vi "Dashboard Main.vi"() -> ()   [LabVIEW 2012]
uses:
  <vilib>/Utility/miscctls.llb/LVRectTypeDef.ctl
  <vilib>/event_ctls.llb/eventvkey.ctl
  <vilib>/Utility/config.llb/Read Key (String).vi
  <vilib>/Utility/config.llb/Read Key (I32).vi
  <vilib>/Utility/config.llb/Write Key (String).vi
  <vilib>/Utility/config.llb/Write Key (I32).vi
  <vilib>/Rock Robotics/Network Tables/SD Write Number.vi
  <vilib>/Rock Robotics/Network Tables/SD Read Number.vi
  <vilib>/Rock Robotics/Network Tables/SD Read Boolean.vi
  <vilib>/Utility/config.llb/NI_LVConfig.lvlib
panel:
  out "Predicted Y Coordionates":sgl
  in  "Camera Settings":T1={"Frate Rate"=10, "Compression"=39, "Size"=1} {"Frate Rate" scale=1.0..30.0; "Size" items=["640x480", "320x240", "160x120"]}
  out "Mode":T2(ring)=enum.""
  out "Camera IP":string="0.0.0.11"
  in  "Dashboard Tab":T3(tab)=enum."Normal Operation"
  out "High Y":dbl
  in  "Red or Hue":cluster{"Lower value":i32, "Upper value":i32}={"Lower value"=52, "Upper value"=255}
  in  "Green or Sat":cluster{"Lower value":i32, "Upper value":i32}={"Lower value"=80, "Upper value"=255}
  in  "Blue or Luma or Val or Inten":cluster{"Lower value":i32, "Upper value":i32}={"Lower value"=80, "Upper value"=255}
  in  "Turn On Vision":bool=TRUE
  out "Vision Working?":bool=TRUE
  out "High Y String":string
  out "Predicted X":sgl
  in  "Crosshair":bool=TRUE
  out "Camera Image 2":T4(plugin-control)
  out "Lines (Shape Detection 1)":T5(array[cluster]) {"End Point"."Y" format="%.2f"; "End Point"."X" format="%.2f"; "Start Point"."Y" format="%.2f"; "Start Point"."X" format="%.2f"}
  in  "Assisted Vision":bool=TRUE
  in  "Blackout":bool=TRUE
  in  "Slider":dbl(slide) scale=0.0..100.0 scale format="%#_3g"
  in  "On/Off":bool caption="Solenoid"
  in  "Test Name":u16(ring) items=["Select the test to run...", "Example Test", "-------------------------------", "List of tests is built in robot code.", "Replace with your own automated tests."]
  in  "Test Tree":string(tree)
  in  "Motor":cluster{"Value":dbl, "Enable":bool} {"Value" scale=-1.0..1.0 scale format="%#_3g"}
  out "Progress":T6 {"Test Progress" scale=0.0..100.0}
  in  "Rev/Fwd":cluster{"Forward":bool, "Reverse":bool}
  in  "Ring":u16(ring) items=["Auto", "Fixed indoor", "Fixed outdoor 1", "Fixed outdoor 2", "Fixed fluorescent 1", "Fixed fluorescent 2", "Hold current"]
  in  "Listbox":i32(listbox)
  out "MotorSlide4":dbl(slide) scale=-1.0..1.0 scale format="%#_2e"
  out "MotorSlide3":dbl(slide) scale=-1.0..1.0 scale format="%#_2e"
  out "MotorSlide2":dbl(slide) scale=-1.0..1.0 scale format="%#_2e"
  in  "MotorName3":string="Front Left"
  in  "MotorName4":string="Front Right"
  in  "MotorName1":string="Rear Left"
  in  "MotorName2":string="Rear Right"
  out "MotorChart4":dbl(graph)
  out "MotorChart3":dbl(graph)
  out "MotorChart2":dbl(graph)
  out "MotorSlide1":dbl(slide) scale=-1.0..1.0 scale format="%#_2e"
  out "MotorChart1":dbl(graph)
  out "JS1 Z":dbl(slide) scale=-1.0..1.0 scale format="%#_2e"
  out "JS2 Z":dbl(slide) scale=-1.0..1.0 scale format="%#_2e"
  out "Joystick 1":cluster{"X":dbl, "Y":dbl}[](graph)
  out "Joystick 2":cluster{"X":dbl, "Y":dbl}[](graph)
  out "JS Buttons 1":T7
  out "JS Buttons 2":T7
  out "Robot IP":string="0.0.0.0"
  out "Battery Value":dbl(slide) scale=0.0..14.0 scale format="%#_2e"
  out "Battery":sgl(graph)
  out "Vision Locked On":bool
  out "Upper LED":bool
  out "Lower LED":bool
  out "Shooter RPM":dbl(slide) scale=0.0..12000.0
  out "Shooter Rotation Angle":dbl(knob) scale=0.0..90.0
  out "Up to Speed?":bool
  out "SHOOT!":bool
  out "Angle":dbl
  in  "Viewer":T8(tab)
  out "Mbps":dbl format="%#.1g"
  in  "Enable":bool=TRUE
  in  "DB Camera Config":bool
  out "Mbps":bool
  out "fps":dbl format="%#.1g"
  out "Image Error Message":string="Timeout in Camera Communications"
  out "Camera Image":T4(plugin-control)
  out "Camera Image 3":T4(plugin-control)
  out "Buttons 1":cluster{"1":bool, "2":bool, "3":bool}
  out "Kinect 1":cluster{"X":dbl, "Y":dbl, "Z":dbl} {"X" scale=1.0..-1.0; "Y" scale=1.0..-1.0; "Z" scale=1.0..-1.0}
  out "Buttons 2":cluster{"1":bool, "2":bool, "3":bool}
  out "Kinect 2":cluster{"X":dbl, "Y":dbl, "Z":dbl} {"X" scale=1.0..-1.0; "Y" scale=1.0..-1.0; "Z" scale=1.0..-1.0}
  out "Version":string
  out "Skeleton Picture":picture
  out "Players":i8
  out "Tree":string(tree)
  # "http://team223.com/Images/TopPane/spinning-gear.gif"
  # "Drive & Motors"
  # "Robot IP:"
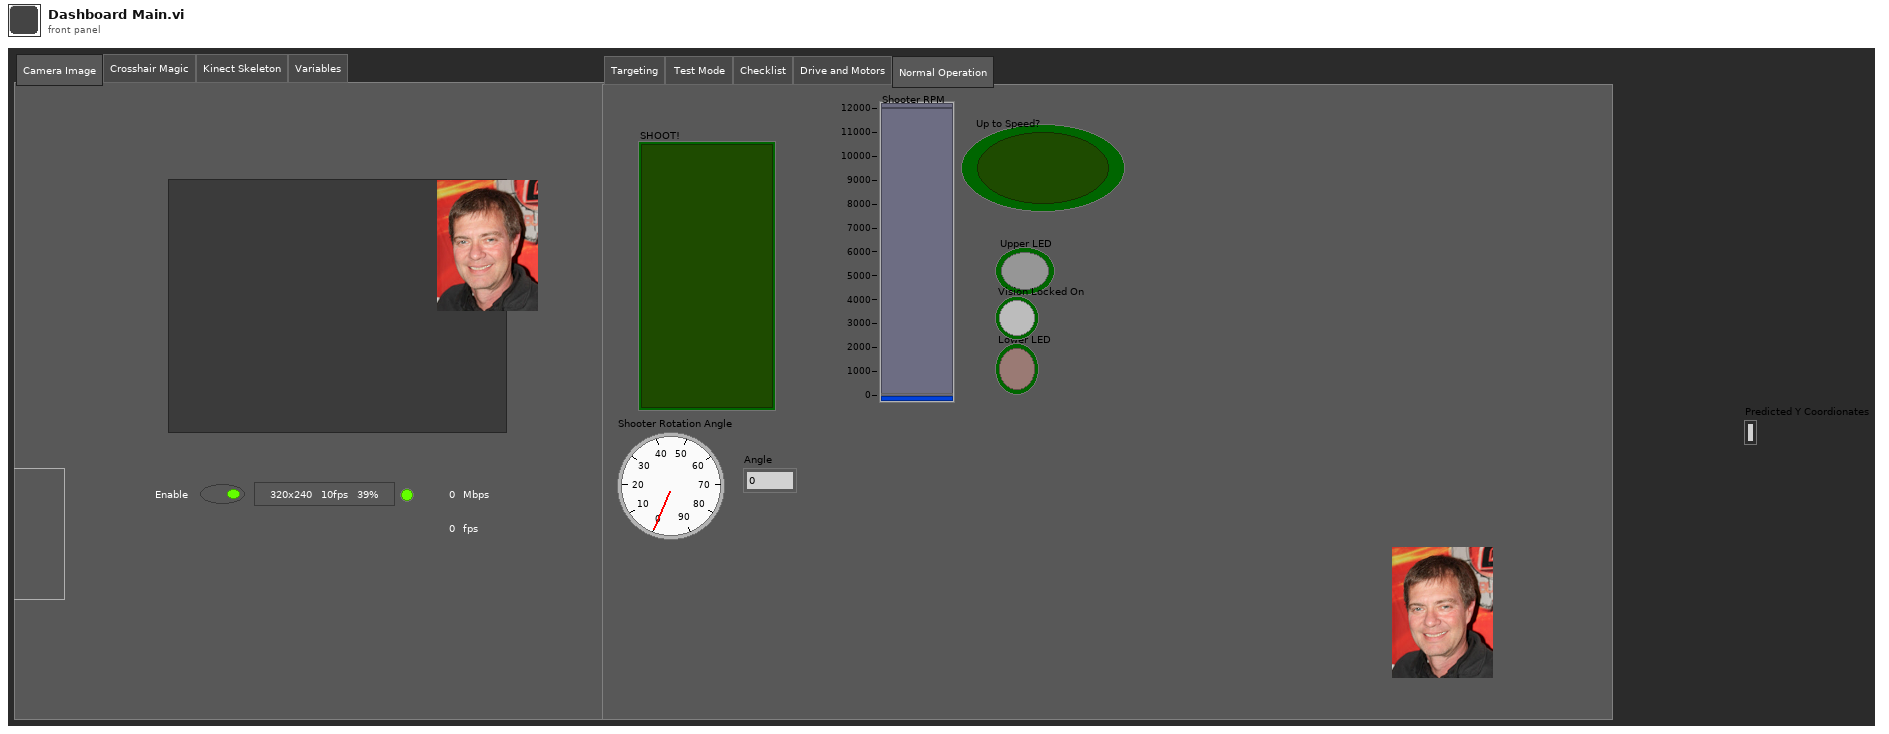
[diagram p1: front panel]
types:
  T1 = cluster{"Frate Rate":i32, "Compression":i32, "Size":u16}
  T2 = enum8{"Tele-Op Disabled", "Tele-Op Enabled", "Auto Disabled", "Auto Enabled", "Test Disabled", "Test Enabled", ""}
  T3 = enum32{"Targeting", "Test Mode ", "Checklist", "Drive and Motors", "Normal Operation"}
  T4 = typedef "IMAQ Image.ctl" = refnum<image>
  T5 = cluster{"Start Point":cluster{"X":sgl, "Y":sgl}, "End Point":cluster{"X":sgl, "Y":sgl}, "Length":dbl, "Orientation":dbl, "Score":dbl}[]
  T6 = cluster{"Test Progress":u8, "Test Progress Text":string}
  T7 = cluster{bool, bool, bool, bool, bool, bool, bool, bool, bool, bool, bool, bool}
  T8 = enum32{"Camera Image", "Crosshair Magic", "Kinect Skeleton", "Variables"}
  T9 = typedef "Image Type" = u32
  T10 = typedef "LVBoundsTypeDef.ctl" = cluster{"Width":u32, "Height":u32}
  T11 = typedef "SkeletonTrackState.ctl" = enum32{"NotTracked", "PositionOnly", "Tracked"}
  T12 = cluster{"TrackingState":u8[], "Position":cluster{"x":sgl, "y":sgl, "z":sgl}, cluster{"x":sgl, "y":sgl, "z":sgl, sgl}[], "TrackState":T11}
  T13 = cluster{cluster{"ScaledToPercentRange":dbl, "ScaledToPercentRange":dbl, "ScaledToPercentRange":dbl}, cluster{bool, bool, bool}}[]
  T14 = cluster{cluster{"ScaledToPercentRange":dbl, "ScaledToPercentRange":dbl, "ScaledToPercentRange":dbl}, cluster{bool, bool, bool}}
  T15 = cluster{"ScaledToPercentRange":dbl, "ScaledToPercentRange":dbl, "ScaledToPercentRange":dbl}
  T16 = typedef "LVRectTypeDef.ctl" = cluster{"Left":i16, "Top":i16, "Right":i16, "Bottom":i16}
  T17 = cluster{"Left":i32, "Top":i32, "Right":i32, "Bottom":i32}
  T18 = cluster{"Competition mode":bool, "Robot Link":bool, "Autonomous":bool, "Enabled":bool, "E-Stop":bool, "Simulated":bool, "TestMode":bool, "Docked Window":bool}
  T19 = cluster{"Boolean Array[0]":bool, "Boolean Array[1]":bool, "Boolean Array[2]":bool, "Boolean Array[3]":bool, "Boolean Array[4]":bool, "Boolean Array[5]":bool, "Boolean Array[6]":bool, "Boolean Array[7]":bool, "Boolean Array[8]":bool, "Boolean Array[9]":bool, "Boolean Array[10]":bool, "Boolean Array[11]":bool}
  T20 = typedef "NI_LVConfig.lvlib/Config Data RefNum.ctl" = refnum<k1>
  T21 = cluster{"Boolean array[0]":bool, "Boolean array[1]":bool, "Boolean array[2]":bool, "Boolean array[3]":bool, "Boolean array[4]":bool, "Boolean array[5]":bool, "Boolean array[6]":bool, "Boolean array[7]":bool, "Boolean array[8]":bool}
  T22 = typedef "eventvkey.ctl" = enum16{"ASCII", "Enter", "Return", "Shift", "Ctrl", "Alt", "Cmd", "Opt", "Caps", "NumLock", "Clear", "Break", "Up", "Down", "Left", "Right", "Insert", "Delete", "Home", "End", "PageUp", "PageDown", "Escape", "Help", "Pause", "ScrollLock", "F1", "F2", "F3", "F4", "F5", "F6", "F7", "F8", "F9", "F10", "F11", "F12", "F13", "F14", "F15", "F16", "F17", "F18", "F19", "F20", "F21", "F22", "F23", "F24", "Play", "VolumeUp", "VolumeDown", "Mute", "Two Byte Char"}
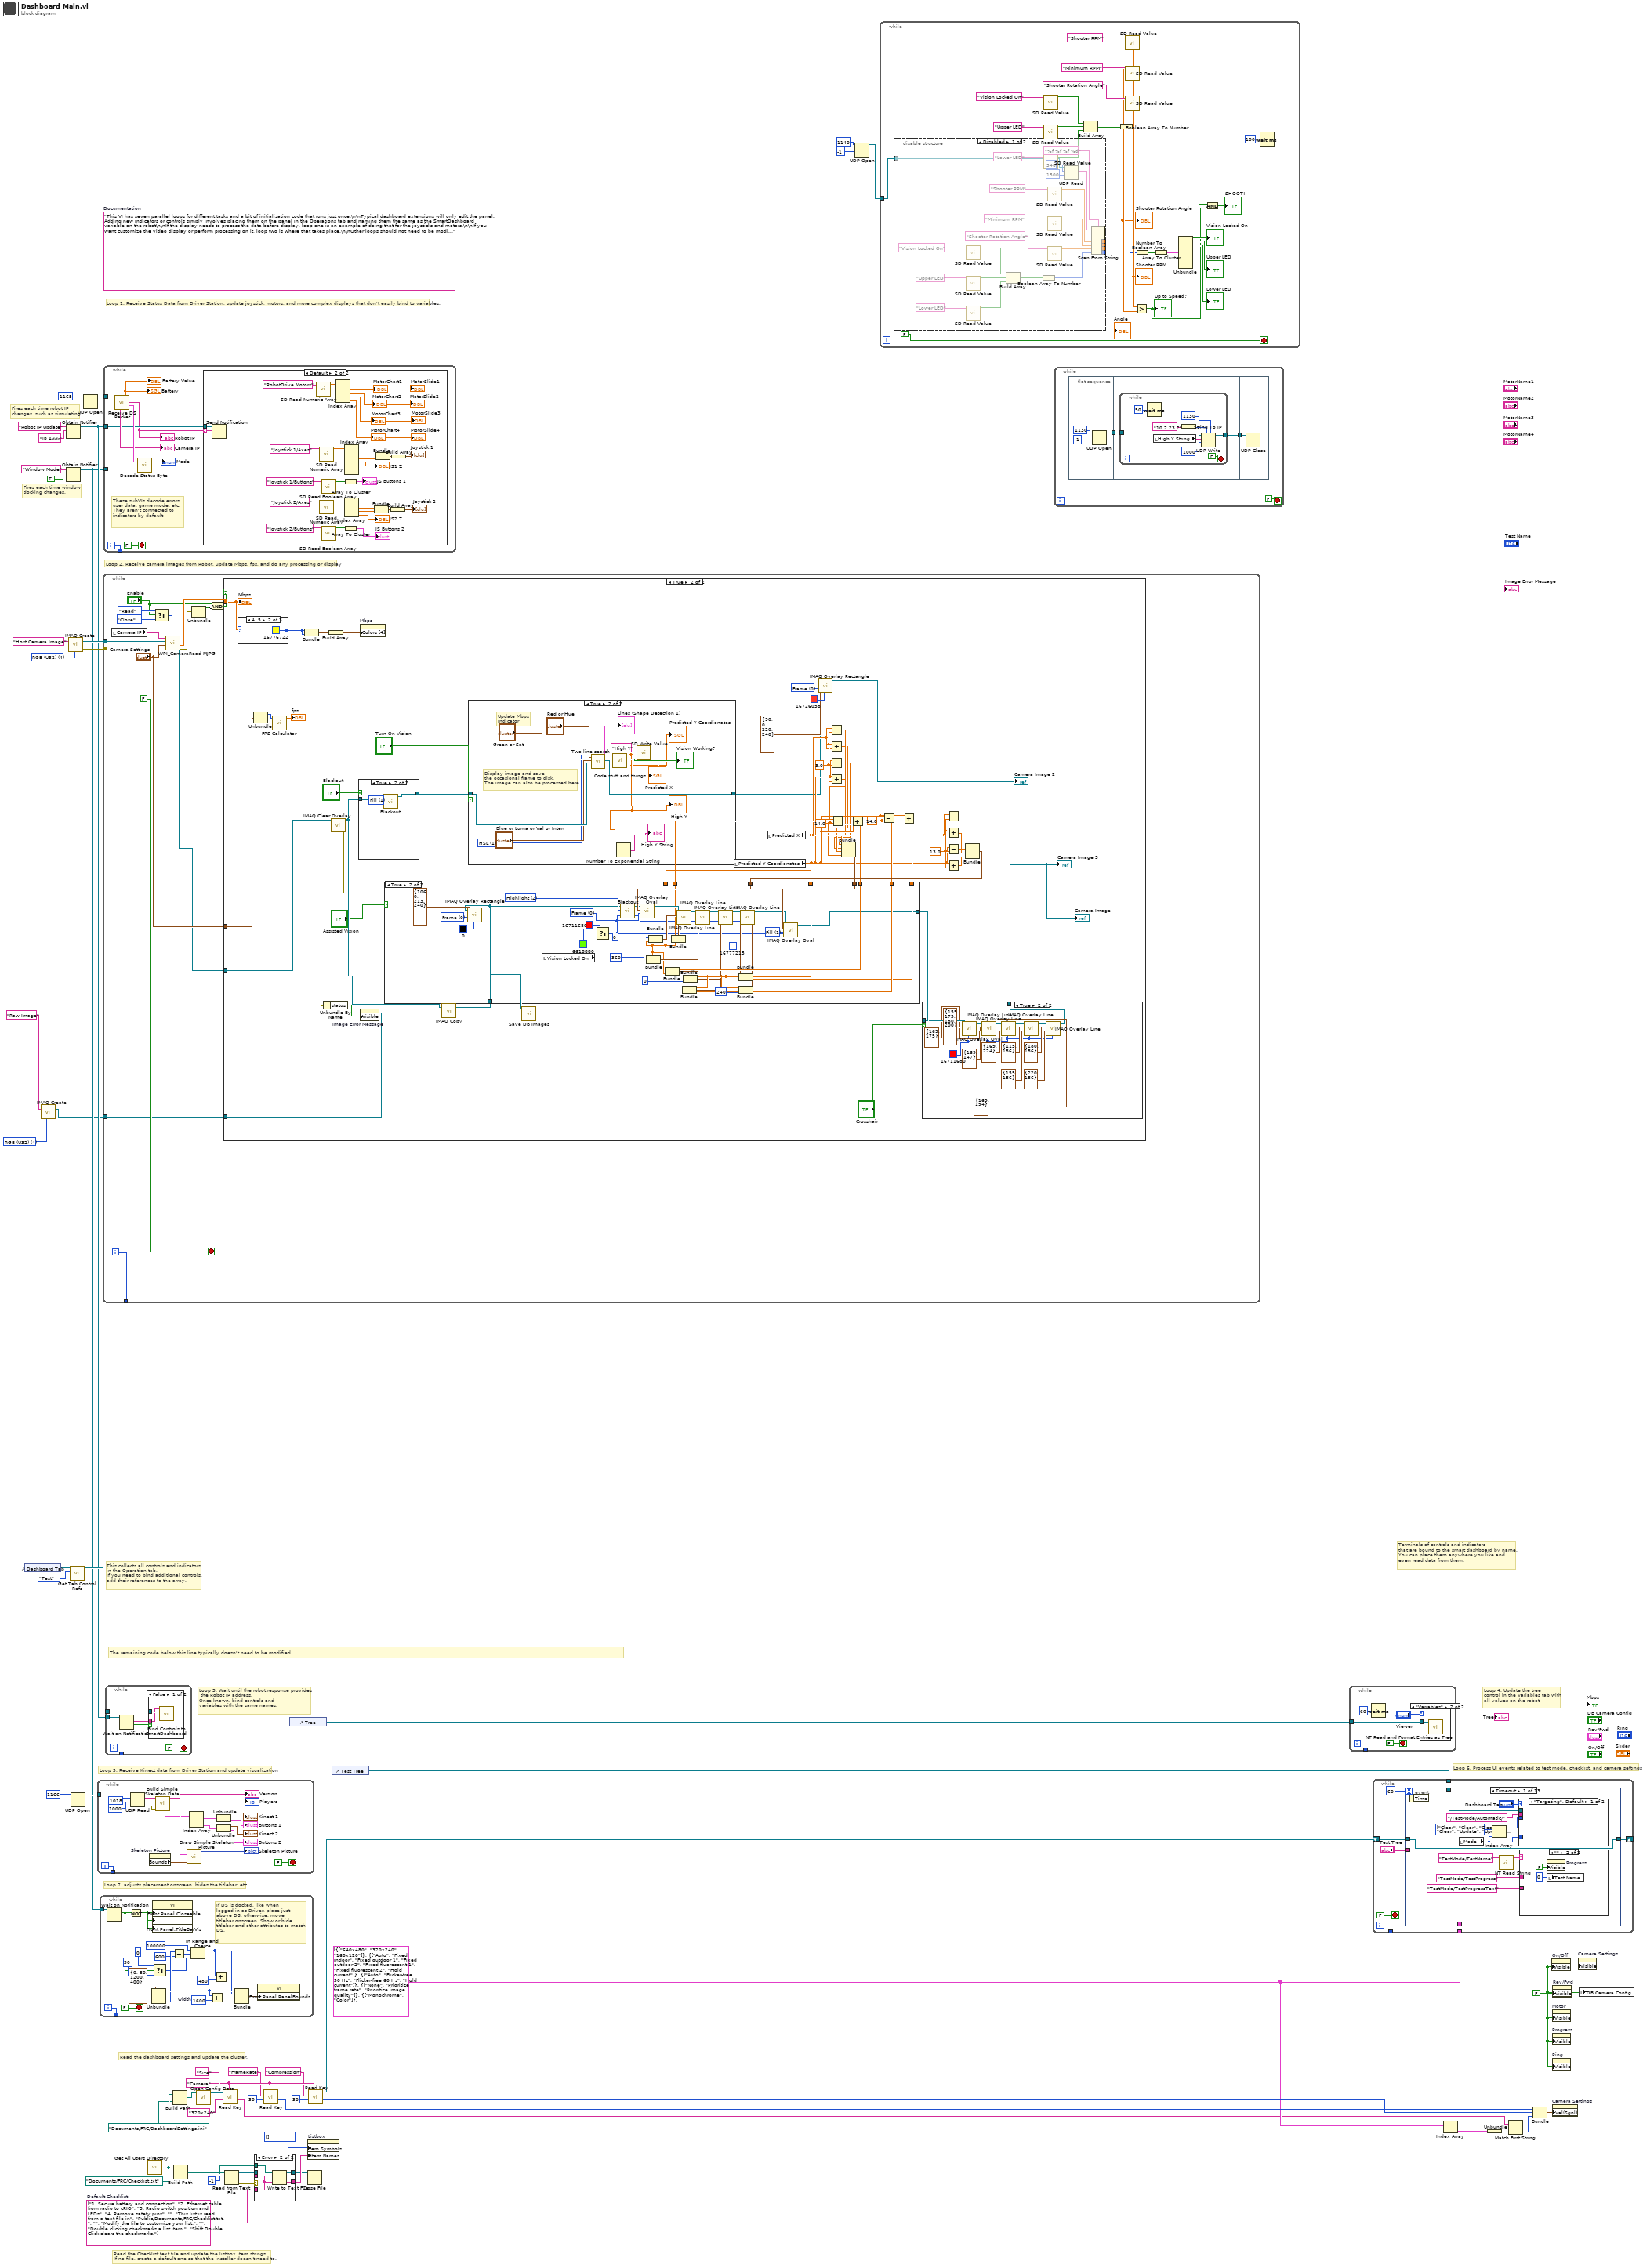
[diagram p0: block diagram]
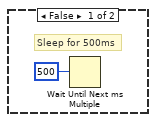
[diagram p4: hidden frame]
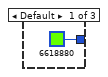
[diagram p9: hidden frame]
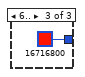
[diagram p10: hidden frame]
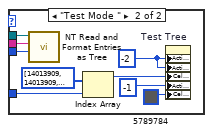
[diagram p12: hidden frame]
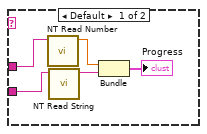
[diagram p13: hidden frame]
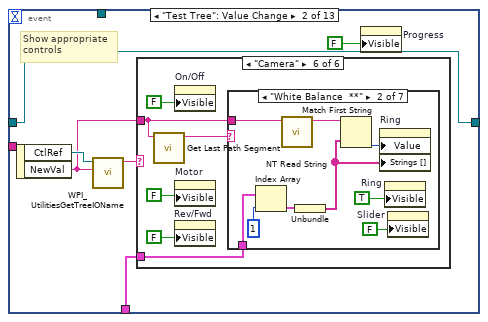
[diagram p14: hidden frame]
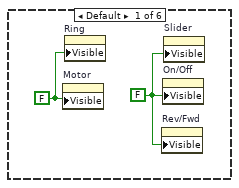
[diagram p15: hidden frame]
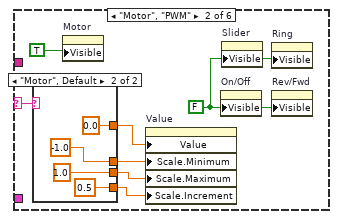
[diagram p16: hidden frame]
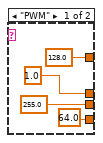
[diagram p17: hidden frame]
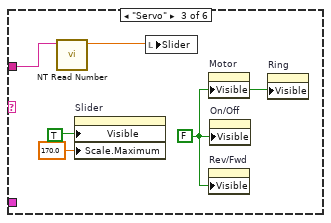
[diagram p18: hidden frame]
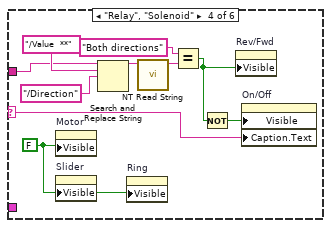
[diagram p19: hidden frame]
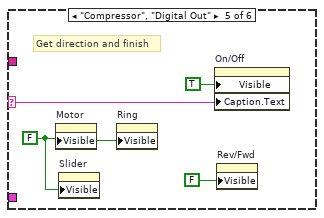
[diagram p20: hidden frame]
diagram:
  w6 = T9 4 items=["Grayscale (U8)", "Grayscale (I16)", "Grayscale (SGL)", "Complex (CSG)", "RGB (U32)", "HSL (U32)", "RGB (U64)"] ("Image Type")
  w27 = "Camera"
  w19 = cluster{string[]}[] [{["640x480", "320x240", "160x120"]}, {["Auto", "Fixed indoor", "Fixed outdoor 1", "Fixed outdoor 2", "Fixed fluorescent 1", "Fixed fluorescent 2", "Hold current"]}, {["Auto", "Flicker-free 50 Hz", "Flicker-free 60 Hz", "Hold current"]}, {["None", "Prioritize frame rate", "Prioritize image quality"]}, {["Monochrome", "Color"]}]
  w35 = string[] ["1. Secure battery and connection", "2. Ethernet cable from radio to cRIO", "3. Radio switch position and LEDs", "4. Remove safety pins", "", "This list is read from a text file in", "Public/Documents/FRC/Checklist.txt.", "", "Modify the file to customize your list.", "", "Double clicking checkmarks a list item.", "Shift Double Click clears the checkmarks."]  # Default Checklist
  w33 = FALSE ("Visible")
  (unwired) "This VI has seven parallel loops for different tasks and a bit of initialization code that runs just once.\n\nTypical dashboard extensions will only edit the panel. Adding new indicators or controls simply involves placing them on the panel in the Operations tab and naming them the same as the SmartDashboard variable on the robot\n\nIf the display needs to process the data before display, loop one is an example of doing that for the joysticks and motors.\n\nIf you want customize the video display or perform processing on it, loop two is where that takes place.\n\nOther loops should not need to be modified. They are pretty standard, and document the task they perform."  # Documentation
  w56 = T9 4 items=["Grayscale (U8)", "Grayscale (I16)", "Grayscale (SGL)", "Complex (CSG)", "RGB (U32)", "HSL (U32)", "RGB (U64)"] ("Image Type")
  # "Fires each time robot IP\nchanges, such as simulating"
  # "Fires each time window\ndocking changes."
  # "Read the Checklist text file and update the listbox item strings.\nIf no file, create a default one so that the installer doesn't need to."
  # "This collects all controls and indicators\nin the Operation tab.\nIf you need to bind additional controls,\nadd their references to the array."
  # "The remaining code below this line typically doesn't need to be modified."
  # "Loop 6. Process UI events related to test mode, checklist, and camera settings"
  # "Read the dashboard settings and update the cluster."
  # "Terminals of controls and indicators\nthat are bound to the smart dashboard by name.\nYou can place them anywhere you like and\neven read data from them."
  # "Loop 4. Update the tree\ncontrol in the Variables tab with\nall values on the robot"
  # "Loop 3. Wait until the robot response provides\n the Robot IP address.\nOnce known, bind controls and\nvariables with the same names."
  # "Loop 5. Receive Kinect data from Driver Station and update visualization"
  # "Loop 7. adjusts placement onscreen, hides the titlebar, etc."
  # "Loop 1. Receive Status Data from Driver Station, update joystick, motors, and more complex displays that don't easily bind to variables."
  # "Loop 2. Receive camera images from Robot, update Mbps, fps, and do any processing or display"
  n1 = control-ref of="Dashboard Tab"() -> (w49:refnum<vi>)
  n2 = call "IMAQ Create"("Image Name"="Raw Image", "Image Type"=w6) -> ("New Image"=w4:T4)  [unwired: 2 in, 2 out]
  n3 = Obtain Notifier(name (unnamed)="Robot IP Update", notification data type="IP Addr" ("name (unnamed)")) -> (notifier out=w46:refnum<notifier>)  [unwired: 2 in, 2 out]
  n4 = Obtain Notifier(name (unnamed)="Window Mode", notification data type=TRUE) -> (notifier out=w39:refnum<notifier>)  [unwired: 2 in, 2 out]
  n5 = call "IMAQ Create"("Image Name"="Host Camera Image", "Image Type"=w56) -> ("New Image"=w54:T4, "error out"=w53:errorcluster)  [unwired: 2 in, 1 out]
  n6 = call <vilib>:"Get Tab Control Refs.vi"("Page Index"=enum32{"Operation", "Test"}."Test" ("Dashboard Tab"), "TabControl in"=w49) -> ("ControlsOnPage"=w50:refnum<vi>[])  [unwired: 9 in]
  n7 = UDP Open(11:u16 1166 ("port")) -> (port=w51:refnum<k16>)  [unwired: 2 in, 4 out]
  n8 = UDP Open(11:u16 1165 ("port")) -> (port=w57:refnum<k16>)  [unwired: 2 in, 4 out]
  n9 = while {
    tunnel: w51 -> [w75]
    tunnel: [w60] -> _
    i -> [w60]
    stop <- FALSE stop-if-true
    n10 = UDP Read(connection ID=w75, max size (548)=1018 ("bytes to read"), timeout ms (25000)=1000) -> (data out=w69:string, error out=w59:errorcluster)  [unwired: 1 in, 3 out]
    n11 = property on="Skeleton Picture" class="Pict"() -> ("Bounds"=w71:T10)  [unwired: 2 in, 2 out]
    n12 = call "Build Simple Skeleton Data.vi"("error in (no error)"=w59, "data in"=w69) -> ("Skeleton Data"=w70:T12, "NumPlayers"=→"Players":i8, "Version String"=→"Version":string, "Simple Joystick Info"=w67:T13)  [unwired: 5 in, 1 out]
    n13 = call "Draw Simple Skeleton Picture.vi"("Bounds"=w71, "Simple Skeleton"=w70) -> ("new picture out"=→"Skeleton Picture":picture)  [unwired: 9 in]
    n14 = Index Array(array=w67) -> (element #1=w66:T14, element #2=w65:T14)  [unwired: 2 in]
    n15 = Unbundle(w66) -> (→"Kinect 1":T15, →"Buttons 1":cluster{bool, bool, bool})
    n16 = Unbundle(w65) -> (→"Kinect 2":T15, →"Buttons 2":cluster{bool, bool, bool})
  }
  n17 = while {
    tunnel: w39 -> [w96]
    tunnel: [w94] -> _
    i -> [w94]
    stop <- FALSE stop-if-true
    w87 = 1600  # width
    # "If DS is docked, like when\nlogged in as Driver, place just\nabove DS, otherwise, move\ntitlebar onscreen. Show or hide\ntitlebar and other attributes to match\nDS."
    n18 = Wait on Notification(notifier=w96) -> (notification=w82:bool)  [unwired: 3 in, 3 out]
    n19 = Not(x=w82) -> (.not. x?=w95:bool)
    n20 = Unbundle(T16 {"Left"=0, "Top"=80, "Right"=1200, "Bottom"=400} ("cluster")) -> ("Left"=w91:i16, "Bottom"=w88:i16)  [unwired: 2 out]
    n21 = property class="VI"("Front Panel.Closeable"=w95, "Front Panel.Minimizeable"=w95, "Front Panel.TitleBarVis"=w95) -> ()  [unwired: 2 in, 2 out]
    n22 = Select(t=0, s=w82, f=30) -> (s? t:f=w81:i32)
    n23 = Subtract(x=w88, y=600) -> (x-y=w85:i32)
    n24 = In Range and Coerce(upper limit=100000, x=w85, lower limit=w81) -> (coerced(x)=w79:i32)  [unwired: 1 out]
    n25 = Add(x=w91, y=w87) -> (x+y=w92:i32)
    n26 = Add(x=w79, y=480 ("height")) -> (x+y=w89:i32)
    n27 = Bundle("Left"=w91, w79, w92, w89) -> (w93:cluster{"Left":i16, i32, i32, i32})  [unwired: 1 out]
    n28 = property class="VI"("Front Panel.PanelBounds"=w93) -> ()  [unwired: 2 in, 2 out]
  }
  n29 = while {
    tunnel: w54 -> [w108]
    tunnel: w53 -> [_]
    tunnel: [w111] -> _
    tunnel: w4 -> [w98]
    i -> [w111]
    stop <- FALSE stop-if-true
    n30 = local read "Camera IP"() -> (w110:string)
    n31 = Select(t=enum16{"Read", "Reopen", "Close"}."Read" ("Operation"), s="Enable", f=enum16{"Read", "Reopen", "Close"}."Close" ("Operation")) -> (s? t:f=w103:enum16{"Read", "Reopen", "Close"})
    n32 = call <vilib>:"WPI_CameraRead MJPG.vi"("Operation"=w103, "Camera Settings"="Camera Settings", "Image"=w108, "address"=w110) -> ("error out"=w102:errorcluster, "Bandwidth (kbps)"=w106:dbl, "Image Out"=w107:T4)  [unwired: 5 in]
    n33 = Unbundle(w102) -> ("status"=w100:bool)  [unwired: 2 out]
    n34 = Compound Arithmetic op=AND("Enable", invert w100) -> (w99:bool)
    n35 = case shown="True" w99 {
      tunnel: "Camera Settings" -> [_ w150]
      tunnel: w107 -> [_ w153]
      tunnel: w106 -> [_ w152]
      tunnel: w98 -> [_ w148]
      frame False {
        # "Sleep for 500ms"
        n36 = Wait Until Next ms Multiple(millisecond multiple=u32 500) -> ()  [unwired: 1 out]
      }
      frame True {
        w121 = u32 0 items=["Frame", "Fill", "Highlight"] ("Drawing Mode (Frame)")
        w129 = 3.0 ("x")
        w132 = sgl 14.0 ("y")
        w134 = sgl 14.0 ("y")
        w144 = 13.0 ("x")
        # "Update Mbps\nindicator"
        n37 = case shown="4, 5" w152 {
          tunnel: [u32 6618880 ("Color Box") u32 16776722 ("Color Box") u32 16716800 ("Color Box")] -> w154
          frame Default {
          }
          frame 4, 5 {
          }
          frame 6.. {
          }
        }
        n38 = Unbundle(w150) -> ("Frate Rate"=w149:i32)  [unwired: 2 out]
        n39 = call "FPS Calculator.vi"("Average Count"=w149) -> ("fps"=→"fps":dbl)  [unwired: 10 in]
        n40 = Bundle("Color Box"=w154, "Color Box"=w154) -> (w156:cluster{"Color Box":u32, "Color Box":u32})  [unwired: 1 out]
        n41 = Build Array(w156) -> (w155:cluster{"Color Box":u32, "Color Box":u32}[])
        n42 = call "IMAQ Clear Overlay"("Image"=w153) -> ("error out"=w157:errorcluster, "Image Out"=w147:T4)  [unwired: 2 in, 7 out]
        n43 = Unbundle By Name(w157) -> ("status"=w158:bool)
        n44 = case shown="True" "Blackout" {
          tunnel: w147 -> [w176 w179]
          tunnel: [w176 w178] -> w146
          frame False {
          }
          frame True {
            w177 = u32 1 items=["Frame", "Fill", "Highlight"] ("Drawing Mode (Frame)")
            n45 = call "Blackout.vi"("Drawing Mode (Frame)"=w177, "Image"=w179) -> ("Image Out"=w178:T4)  [unwired: 9 in]
          }
        }
        n46 = property on="Mbps" class="Bool (strict)"("Colors [4]"=w155) -> ()  [unwired: 2 in, 2 out]
        n47 = property on="Image Error Message" class="Str"("Visible"=w158) -> ()  [unwired: 2 in, 2 out]
        n48 = call "IMAQ Copy"("Image Dst"=w148, "Image Src"=w147) -> ("Image Dst Out"=w145:T4)  [unwired: 4 in, 1 out]
        n49 = case shown="True" "Turn On Vision" {
          tunnel: w146 -> [w219 w232]
          tunnel: [w219 w231] -> w119
          frame False {
          }
          frame True {
            w226 = u16 1 items=["RGB", "HSL", "HSV", "HSI"] ("Color Mode (Color Threshold 1)")
            # "Display image and save\nthe occasional frame to disk.\nThe image can also be processed here."
            n50 = call "Two line search.vi"("Color Mode (Color Threshold 1)"=w226, "Red or Hue Range (Color Threshold 1)"="Red or Hue", "Green or Sat Range (Color Threshold 1)"="Green or Sat", "Blue or Luma or Val or Inten Range (Color Threshold 1)"="Blue or Luma or Val or Inten", "Camera Image 3"=w232) -> ("Lines (Shape Detection 1)"=w225:T5, "Image Out"=w231:T4)  [unwired: 18 in, 3 out]
            "Lines (Shape Detection 1)" <- w225
            n51 = call "Code stuff and things.vi"("Lines (Shape Detection 1) in"=w225) -> ("Predicted Y Coordinates"=→"Predicted Y Coordionates":sgl, "Predicted X Coordinates"=→"Predicted X":sgl, "Dun Fuk Up?"=→"Vision Working?":bool, "Chosen Y"=w223:sgl)  [unwired: 7 in]
            "High Y" <- w223
            n52 = Number To Exponential String(number=w223) -> (E-format string=→"High Y String":string)  [unwired: 3 in]
            n53 = call-poly <vilib>:"SD Write Value.vi"("Numeric"=w223, "Name"="High Y") -> ()  [unwired: 8 in, 2 out]
          }
        }
        n54 = call "Save DB Images.vi"("Image"=w145) -> ()  [unwired: 2 in, 1 out]
        n55 = local read "Predicted Y Coordionates"() -> (w127:sgl)
        n56 = local read "Predicted X"() -> (w128:sgl)
        n57 = call "IMAQ Overlay Rectangle"("Color"=u32 16726058, "Drawing Mode (Frame)"=w121, "Rectangle"=T17 {"Left"=90, "Top"=0, "Right"=220, "Bottom"=240}, "Image"=w119) -> ("Image Out"=→"Camera Image 2":T4)  [unwired: 2 in, 5 out]
        n58 = Subtract(x=w128, y=w129) -> (x-y=w126:dbl)
        n59 = Add(x=w129, y=w128) -> (x+y=w125:dbl)
        n60 = Subtract(x=w127, y=w129) -> (x-y=w124:dbl)
        n61 = Add(x=w127, y=w129) -> (x+y=w123:dbl)
        n62 = Subtract(x=w128, y=w134) -> (x-y=w135:sgl)
        n63 = Bundle(w126, w124, w125, w123) -> (w138:cluster{dbl, dbl, dbl, dbl})  [unwired: 1 in]
        n64 = Add(x=w128, y=w134) -> (x+y=w133:sgl)
        n65 = Subtract(x=w127, y=w132) -> (x-y=w131:sgl)
        n66 = Add(x=w127, y=w132) -> (x+y=w130:sgl)
        n67 = Subtract(x=w128, y=w144) -> (x-y=w143:dbl)
        n68 = Add(x=w144, y=w128) -> (x+y=w141:dbl)
        n69 = Subtract(x=w127, y=w144) -> (x-y=w142:dbl)
        n70 = Add(x=w127, y=w144) -> (x+y=w140:dbl)
        n71 = Bundle(w143, w142, w141, w140) -> (w139:cluster{dbl, dbl, dbl, dbl})  [unwired: 1 in]
        n72 = case shown="True" "Assisted Vision" {
          tunnel: w145 -> [w180 w214]
          tunnel: [w180 w186] -> w136
          tunnel: w139 -> [_ w213]
          tunnel: w138 -> [_ w188]
          tunnel: w127 -> [_ w200]
          tunnel: w135 -> [_ w204]
          tunnel: w133 -> [_ w199]
          tunnel: w128 -> [_ w196]
          tunnel: w131 -> [_ w195]
          tunnel: w130 -> [_ w194]
          frame False {
          }
          frame True {
            w185 = u32 1 items=["Frame", "Fill"] ("Drawing Mode (Frame)")
            (unwired) u32 16777215 ("BG Color (Transparent)")
            w211 = u32 0 items=["Frame", "Fill", "Highlight"] ("Drawing Mode (Frame)")
            w215 = u32 2 items=["Frame", "Fill", "Highlight"] ("Drawing Mode (Frame)")
            w217 = u32 0 items=["Frame", "Fill", "Highlight"] ("Drawing Mode (Frame)")
            n73 = call "IMAQ Overlay Rectangle"("Color"=u32 0, "Drawing Mode (Frame)"=w217, "Rectangle"=T17 {"Left"=106, "Top"=0, "Right"=213, "Bottom"=240}, "Image"=w214) -> ()  [unwired: 2 in, 6 out]
            n74 = local read "Vision Locked On"() -> (w183:bool)
            n75 = Select(t=u32 6618880, s=w183, f=u32 16711680 ("Color")) -> (s? t:f=w184:u32)
            n76 = call "Blackout.vi"("Drawing Mode (Frame)"=w215, "Image"=w214) -> ("Image Out"=w212:T4)  [unwired: 9 in]
            n77 = call "IMAQ Overlay Oval"("Color"=w184, "Drawing Mode (Frame)"=w211, "Bounding Rectangle"=w213, "Image"=w212) -> ("Image Out"=w207:T4)  [unwired: 6 in, 1 out]
            n78 = Bundle("X"=360, "Predicted Y Coordionates"=w200) -> (w201:cluster{"X":i32, "Predicted Y Coordionates":sgl})  [unwired: 1 in]
            n79 = Bundle("X"=0, "Predicted Y Coordionates"=w200) -> (w205:cluster{"X":i32, "Predicted Y Coordionates":sgl})  [unwired: 1 in]
            n80 = Bundle(w199, "Predicted Y Coordionates"=w200) -> (w189:cluster{sgl, "Predicted Y Coordionates":sgl})  [unwired: 1 in]
            n81 = Bundle(w204, "Predicted Y Coordionates"=w200) -> (w203:cluster{sgl, "Predicted Y Coordionates":sgl})  [unwired: 1 in]
            n82 = call "IMAQ Overlay Line"("Color"=w184, "End Point"=w203, "Start Point"=w205, "Image"=w207) -> ("Image Out"=w210:T4)  [unwired: 6 in, 1 out]
            n83 = Bundle("Predicted X"=w196, w195) -> (w192:cluster{"Predicted X":sgl, sgl})  [unwired: 1 in]
            n84 = Bundle("Predicted X"=w196, "X"=0) -> (w193:cluster{"Predicted X":sgl, "X":i32})  [unwired: 1 in]
            n85 = call "IMAQ Overlay Line"("Color"=w184, "End Point"=w201, "Start Point"=w189, "Image"=w210) -> ("Image Out"=w209:T4)  [unwired: 6 in, 1 out]
            n86 = call "IMAQ Overlay Line"("Color"=w184, "End Point"=w192, "Start Point"=w193, "Image"=w209) -> ("Image Out"=w208:T4)  [unwired: 6 in, 1 out]
            n87 = Bundle("Predicted X"=w196, w194) -> (w191:cluster{"Predicted X":sgl, sgl})  [unwired: 1 in]
            n88 = Bundle("Predicted X"=w196, "X"=240) -> (w190:cluster{"Predicted X":sgl, "X":i32})  [unwired: 1 in]
            n89 = call "IMAQ Overlay Line"("Color"=w184, "End Point"=w190, "Start Point"=w191, "Image"=w208) -> ("Image Out"=w187:T4)  [unwired: 6 in, 1 out]
            n90 = call "IMAQ Overlay Oval"("Color"=w184, "Drawing Mode (Frame)"=w185, "Bounding Rectangle"=w188, "Image"=w187) -> ("Image Out"=w186:T4)  [unwired: 6 in, 1 out]
          }
        }
        n91 = case shown="True" "Crosshair" {
          tunnel: w136 -> [w159 w175]
          tunnel: [w159 w161] -> w114
          frame False {
          }
          frame True {
            w160 = u32 16711680 ("Color")
            n92 = call "IMAQ Overlay Oval"("Color"=w160, "Bounding Rectangle"=T17 {"Left"=155, "Top"=175, "Right"=180, "Bottom"=200}, "Image"=w175) -> ("Image Out"=w162:T4)  [unwired: 7 in, 1 out]
            n93 = call "IMAQ Overlay Line"("Color"=w160, "End Point"=cluster{"X":i32, "Y":i32} {"X"=169, "Y"=175}, "Start Point"=cluster{"X":i32, "Y":i32} {"X"=169, "Y"=147}, "Image"=w162) -> ("Image Out"=w171:T4)  [unwired: 6 in, 1 out]
            n94 = call "IMAQ Overlay Line"("Color"=w160, "End Point"=cluster{"X":i32, "Y":i32} {"X"=169, "Y"=224}, "Start Point"=cluster{"X":i32, "Y":i32} {"X"=169, "Y"=194}, "Image"=w171) -> ("Image Out"=w172:T4)  [unwired: 6 in, 1 out]
            n95 = call "IMAQ Overlay Line"("Color"=w160, "End Point"=cluster{"X":i32, "Y":i32} {"X"=155, "Y"=186}, "Start Point"=cluster{"X":i32, "Y":i32} {"X"=115, "Y"=186}, "Image"=w172) -> ("Image Out"=w173:T4)  [unwired: 6 in, 1 out]
            n96 = call "IMAQ Overlay Line"("Color"=w160, "End Point"=cluster{"X":i32, "Y":i32} {"X"=220, "Y"=186}, "Start Point"=cluster{"X":i32, "Y":i32} {"X"=180, "Y"=186}, "Image"=w173) -> ("Image Out"=w161:T4)  [unwired: 6 in, 1 out]
          }
        }
        "Camera Image 3" <- w114
        "Camera Image" <- w114
        "Mbps" <- w152
      }
    }
  }
  n97 = while {
    tunnel: w57 -> [w243]
    tunnel: w46 -> [w237]
    tunnel: w39 -> [w241]
    tunnel: [w238] -> _
    i -> [w238]
    stop <- FALSE stop-if-true
    # "These subVIs decode errors, user data, game mode, etc.\nThey aren't connected to indicators by default"
    n98 = call "Receive DS Packet.vi"("Recv Socket"=w243) -> ("Battery"=→"Battery" →"Battery Value":sgl, "Robot IP Address"=w236:string, "Status"=w244:T18, "Camera IP Address"=→"Camera IP":string)  [unwired: 1 in, 10 out]
    "Robot IP" <- w236
    n99 = call "Decode Status Byte.vi"("Window Mode Notifier"=w241, "Status"=w244) -> ("Mode"=→"Mode":T2)  [unwired: 1 out]
    n100 = case shown="Default" w236 {
      selector: w236 -> [_ w246]
      tunnel: w237 -> [_ w247]
      frame "0.0.0.0" {
        # "Robot not responding, don't poll the variables"
      }
      frame Default {
        n101 = Send Notification(notification=w246, notifier=w247) -> ()  [unwired: 1 in, 2 out]
        n102 = call <vilib>:"SD Read Numeric Array.vi"("Name"="RobotDrive Motors") -> ("Numeric Array"=w270:dbl[])  [unwired: 8 in, 2 out]
        n103 = call <vilib>:"SD Read Numeric Array.vi"("Name"="Joystick 1/Axes") -> ("Numeric Array"=w263:dbl[])  [unwired: 8 in, 2 out]
        n104 = call <vilib>:"SD Read Numeric Array.vi"("Name"="Joystick 2/Axes") -> ("Numeric Array"=w257:dbl[])  [unwired: 8 in, 2 out]
        n105 = call <vilib>:"SD Read Boolean Array.vi"("Name"="Joystick 1/Buttons") -> ("Boolean Array"=w265:bool[])  [unwired: 8 in, 2 out]
        n106 = call <vilib>:"SD Read Boolean Array.vi"("Name"="Joystick 2/Buttons") -> ("Boolean Array"=w256:bool[])  [unwired: 8 in, 2 out]
        n107 = Index Array(array=w270) -> (element #1=→"MotorChart1" →"MotorSlide1":dbl, element #2=→"MotorSlide2" →"MotorChart2":dbl, element #3=→"MotorChart3" →"MotorSlide3":dbl, element #4=→"MotorChart4" →"MotorSlide4":dbl)  [unwired: 4 in]
        n108 = Array To Cluster(array=w265) -> (cluster=→"JS Buttons 1":T19)
        n109 = Array To Cluster(array=w256) -> (cluster=→"JS Buttons 2":T19)
        n110 = Index Array(array=w263) -> (element #1=w260:dbl, element #2=w261:dbl, element #3=→"JS1 Z":dbl)  [unwired: 6 in, 3 out]
        n111 = Index Array(array=w257) -> (element #1=w252:dbl, element #2=w251:dbl, element #3=→"JS2 Z":dbl)  [unwired: 3 in]
        n112 = Bundle("Numeric"=w252, "Numeric"=w251) -> (w253:cluster{"Numeric":dbl, "Numeric":dbl})  [unwired: 1 in]
        n113 = Bundle("Numeric"=w260, "Numeric"=w261) -> (w259:cluster{"Numeric":dbl, "Numeric":dbl})  [unwired: 1 in]
        n114 = Build Array(w253) -> (→"Joystick 2":cluster{"Numeric":dbl, "Numeric":dbl}[])
        n115 = Build Array(w259) -> (→"Joystick 1":cluster{"Numeric":dbl, "Numeric":dbl}[])
      }
    }
  }
  n116 = while {
    tunnel: w50 -> [w279]
    tunnel: w46 -> [w276]
    tunnel: [w274] -> _
    i -> [w274]
    stop <- FALSE stop-if-true
    n117 = Wait on Notification(notifier=w276) -> (notification=w275:string, timed out?=w277:bool)  [unwired: 3 in, 2 out]
    n118 = case shown="False" w277 {
      tunnel: w279 -> [w281 _]
      tunnel: w275 -> [w280 _]
      frame False {
        n119 = call <vilib>:"Bind Controls to SmartDashboard.vi"("Bound Control Refs"=w281, "Server IP Address"=w280) -> ()  [unwired: 10 in]
      }
      frame True {
      }
    }
  }
  n120 = call "Get All Users Directory.vi"() -> ("All User Path"=w32:path)
  n121 = Build Path(base path=w32, name or relative path=path "Documents/FRC/DashboardSettings.ini") -> (appended path=w31:path)
  n122 = Build Path(base path=w32, name or relative path=path "Documents/FRC/Checklist.txt") -> (appended path=w36:path)
  n123 = call <vilib>:"Open Config Data.vi"("configuration file path"=w31) -> ("refnum"=w30:T20)  [unwired: 8 in, 2 out]
  n124 = call-poly <vilib>:"Read Key.vi"("section"=w27, "default value"="320x240", "key"="Size", "refnum"=w30) -> ("value"=w17:string, "refnum out"=w12:T20)  [unwired: 2 in, 4 out]
  n125 = Read from Text File(file (use dialog)=w36, count=-1 ("timeout ms (25000)")) -> (refnum out=w14:refnum<file>, text=w37:string[], error out=w38:errorcluster)  [unwired: 2 in, 1 out]
  n126 = case shown="Error" w38 {
    tunnel: w37 -> [w283 _]
    tunnel: [w283 w285] -> w34
    tunnel: w35 -> [_ w285]
    tunnel: w36 -> [_ w286]
    tunnel: [w282 w284] -> w13
    tunnel: w14 -> [w282 _]
    frame No Error {
    }
    frame Error {
      n127 = Write to Text File(file (use dialog)=w286, text=w285) -> (refnum out=w284:refnum<file>)  [unwired: 2 in, 2 out]
    }
  }
  n128 = call-poly <vilib>:"Read Key.vi"("section"=w27, "default value"=30, "key"="FrameRate", "refnum"=w12) -> ("value"=w22:i32, "refnum out"=w11:T20)  [unwired: 1 in, 5 out]
  n129 = control-ref of="Tree"() -> (w8:refnum<vi>)
  n130 = property on="Listbox" class="LstBox (strict)"("Item Symbols"=i32[] [], "Item Names"=w34) -> ()  [unwired: 2 in, 2 out]
  n131 = Close File(refnum=w13) -> ()  [unwired: 1 in, 2 out]
  n132 = call-poly <vilib>:"Read Key.vi"("section"=w27, "default value"=30, "key"="Compression", "refnum"=w11) -> ("value"=w21:i32, "refnum out"=w9:T20)  [unwired: 1 in, 5 out]
  n133 = control-ref of="Test Tree"() -> (w7:refnum<vi>)
  n134 = UDP Open(9:-1 ("timeout ms (25000)"), 11:u16 1140 ("port")) -> (port=w2:refnum<k16>)  [unwired: 3 in, 2 out]
  n135 = while {
    tunnel: w2 -> [w310]
    stop <- FALSE stop-if-true
    n136 = disable-structure shown="Disabled" {
      disable-tunnel: w310 -> [w333 _]
      disable-tunnel: [w328 _] -> _
      disable-tunnel: [w327 _] -> _
      disable-tunnel: [w326 _] -> _
      disable-tunnel: [w325 _] -> _
      frame Disabled {
        n137 = call-poly <vilib>:"SD Read Value.vi"("Name"="Vision Locked On") -> ("Boolean"=w315:bool)  [unwired: 8 in, 2 out]
        n138 = call-poly <vilib>:"SD Read Value.vi"("Name"="Upper LED") -> ("Boolean"=w314:bool)  [unwired: 8 in, 2 out]
        n139 = call-poly <vilib>:"SD Read Value.vi"("Name"="Lower LED") -> ("Boolean"=w313:bool)  [unwired: 8 in, 2 out]
        n140 = Build Array(w315, w314, w313) -> (w312:bool[])
        n141 = Boolean Array To Number(Boolean array=w312) -> (number=w311:u32)
        n142 = call-poly <vilib>:"SD Read Value.vi"("Name"="Shooter RPM") -> ("Numeric"=w316:dbl)  [unwired: 8 in, 2 out]
        n143 = call-poly <vilib>:"SD Read Value.vi"("Name"="Minimum RPM") -> ("Numeric"=w317:dbl)  [unwired: 8 in, 2 out]
        n144 = call-poly <vilib>:"SD Read Value.vi"("Name"="Shooter Rotation Angle") -> ("Numeric"=w318:dbl)  [unwired: 8 in, 2 out]
        n145 = UDP Read(connection ID=w333, max size (548)=548, timeout ms (25000)=1500) -> (data out=w330:string)  [unwired: 1 in, 4 out]
        n146 = Scan From String(format string="%f %f %f %d", input string=w330, default 1=w316, default 2=w317, default 3=w318, default 4=w311) -> (output 1=w325:dbl, output 2=w326:dbl, output 3=w327:dbl, output 4=w328:u32)  [unwired: 2 in, 3 out]
      }
      frame Enabled {
      }
    }
    n147 = call-poly <vilib>:"SD Read Value.vi"("Name"="Vision Locked On") -> ("Boolean"=w298:bool)  [unwired: 8 in, 2 out]
    n148 = call-poly <vilib>:"SD Read Value.vi"("Name"="Upper LED") -> ("Boolean"=w299:bool)  [unwired: 8 in, 2 out]
    n149 = call-poly <vilib>:"SD Read Value.vi"("Name"="Lower LED") -> ("Boolean"=w300:bool)  [unwired: 8 in, 2 out]
    n150 = Build Array(w298, w299, w300) -> (w301:bool[])
    n151 = Boolean Array To Number(Boolean array=w301) -> (number=w288:u32)
    n152 = call-poly <vilib>:"SD Read Value.vi"("Name"="Shooter RPM") -> ("Numeric"=w291:dbl)  [unwired: 8 in, 2 out]
    "Shooter RPM" <- w291
    n153 = call-poly <vilib>:"SD Read Value.vi"("Name"="Minimum RPM") -> ("Numeric"=w290:dbl)  [unwired: 8 in, 2 out]
    n154 = call-poly <vilib>:"SD Read Value.vi"("Name"="Shooter Rotation Angle") -> ("Numeric"=→"Shooter Rotation Angle" →"Angle":dbl)  [unwired: 8 in, 2 out]
    n155 = Greater?(x=w291, y=w290) -> (0:w303:bool)
    "Up to Speed?" <- w303
    n156 = Number To Boolean Array(number=w288) -> (Boolean array=w308:bool[])
    n157 = Array To Cluster(array=w308) -> (cluster=w307:T21)
    n158 = Unbundle(w307) -> ("Boolean array[0]"=w304:bool, "Boolean array[1]"=→"Upper LED":bool, "Boolean array[2]"=→"Lower LED":bool)  [unwired: 6 out]
    "Vision Locked On" <- w304
    n159 = And(x=w304, y=w303) -> (x .and. y?=→"SHOOT!":bool)
    n160 = Wait (ms)(milliseconds to wait=u32 100) -> ()  [unwired: 1 out]
  }
  n161 = while {
    stop <- FALSE stop-if-true
    n162 = flat-sequence {
      tunnel: [w337] -> w335
      tunnel: w335 -> [w341]
      tunnel: [w340] -> w334
      tunnel: w334 -> [w351]
      frame #0 {
        n163 = UDP Open(9:-1 ("timeout ms (25000)"), 11:u16 1130 ("port")) -> (port=w337:refnum<k16>)  [unwired: 3 in, 2 out]
      }
      frame #1 {
        n164 = while {
          tunnel: w341 -> [w349]
          tunnel: [w344] -> w340
          stop <- FALSE stop-if-true
          n165 = Wait (ms)(milliseconds to wait=u32 50) -> ()  [unwired: 1 out]
          n166 = local read "High Y String"() -> (w343:string)
          n167 = String To IP(1:"10.2.23.2" ("name")) -> (0:w348:u32)
          n168 = UDP Write(address=w348, port or service name=u16 1130, connection ID=w349, data in=w343, 9:1000 ("timeout ms (25000)")) -> (3:w344:refnum<k16>)  [unwired: 1 in, 1 out]
        }
      }
      frame #2 {
        n169 = UDP Close(connection ID=w351) -> ()  [unwired: 1 in, 2 out]
      }
    }
  }
  n170 = while {
    tunnel: [w353] -> _
    tunnel: w8 -> [w352]
    i -> [w353]
    stop <- FALSE stop-if-true
    n171 = Wait (ms)(milliseconds to wait=u32 60) -> ()  [unwired: 1 out]
    n172 = case shown="\"Variables\"" "Viewer" {
      tunnel: w352 -> [_ w357]
      frame Default {
      }
      frame "Variables" {
        n173 = call <vilib>:"NT Read and Format Entries as Tree.vi"("Tree Refnum"=w357) -> ()  [unwired: 9 in, 2 out]
      }
    }
  }
  n174 = while {
    tunnel: w19 -> [w362]
    shift-right: [w361] -> _
    shift-left: w9 -> [w360]
    tunnel: [w359] -> _
    tunnel: w7 -> [w358]
    i -> [w359]
    stop <- FALSE stop-if-true
    n175 = event shown="[0] Timeout" {
      selector: _ -> [_ _ _ _ _ _ _ _ _ _ _ _ _]
      dyn-events: _ -> [_ _ _ _ _ _ _ _ _ _ _ _ _]
      timeout: u32 60 ("milliseconds to wait") -> [_ _ _ _ _ _ _ _ _ _ _ _ _]
      tunnel: w358 -> [w372 _ _ _ _ _ _ _ _ _ _ _ _]
      tunnel: "Test Tree" -> [_ _ _ _ _ _ _ _ w566 w574 w576 w580 w588]
      tunnel: w362 -> [_ w394 _ _ _ _ w530 w560 _ _ _ _ _]
      tunnel: [w366 w393 _ w496 w504 w516 w529 w553 w565 w572 w575 w579 w587] -> w361
      tunnel: w360 -> [w366 w393 _ w496 w504 w516 w528 w553 w565 w572 w575 w579 w587]
      event Timeout {
        w371 = enum16{"Update", "Clear"}[] [enum."Clear", enum."Clear", enum."Clear", enum."Clear", enum."Update", enum."Update", enum."Clear"] items=["Update", "Clear"]
        n176 = event-data() -> ()  [unwired: 1 in, 1 out]
        n177 = local read "Mode"() -> (w369:T2)
        n178 = Index Array(array=w371, index=w369) -> (element=w370:enum16{"Update", "Clear"})
        n179 = call <vilib>:"NT Read String.vi"("Name"="TestMode/TestName") -> ("String"=w375:string)  [unwired: 9 in, 1 out]
        n180 = case shown="\"Targeting\", Default" "Dashboard Tab" {
          tunnel: w372 -> [_ w385]
          tunnel: "/TestMode/Automatic/" ("Name Pattern") -> [_ w384]
          tunnel: w370 -> [_ w383]
          tunnel: w369 -> [_ w381]
          frame "Targeting", Default {
          }
          frame "Test Mode " {
            w380 = -2 ("Active Item:Row Number")
            n181 = call <vilib>:"NT Read and Format Entries as Tree.vi"("Operation"=w383, "Name Pattern"=w384, "Tree Refnum"=w385) -> ()  [unwired: 7 in, 2 out]
            n182 = Index Array(array=u32[] [14013909, 14013909, 14013909, 14013909, 14013909, 16777215, 14013909], index=w381) -> (element=w379:u32)
            n183 = property on="Test Tree" class="Tree (strict)"("Active Item Row Number"=w380, "ActiveColNum"=w380, "CellBG"=w379, "Active Item Row Number"=-1 ("Active Item:Row Number"), "CellBG"=u32 5789784 ("Color Box")) -> ()  [unwired: 2 in, 2 out]
          }
        }
        n184 = case shown="\"\"" w375 {
          tunnel: "TestMode/TestProgress" ("Name") -> [w387 _]
          tunnel: "TestMode/TestProgressText" ("Name") -> [w386 _]
          frame Default {
            n185 = call <vilib>:"NT Read Number.vi"("Name"=w387) -> ("Numeric"=w388:dbl)  [unwired: 9 in, 1 out]
            n186 = call <vilib>:"NT Read String.vi"("Name"=w386) -> ("String"=w389:string)  [unwired: 9 in, 1 out]
            n187 = Bundle("Numeric"=w388, "String"=w389) -> (→"Progress":cluster{"Numeric":dbl, "String":string})  [unwired: 1 in]
          }
          frame "" {
            n188 = property on="Progress" class="Clust (strict)"("Visible"=FALSE) -> ()  [unwired: 2 in, 2 out]
            n189 = local write "Test Name"(u16 0) -> ()
          }
        }
      }
      event "Test Tree": Value Change {
        # "Show appropriate\ncontrols"
        n190 = event-data() -> ("CtlRef"=w397:refnum<vi>, "NewVal"=w395:string)  [unwired: 1 in]
        n191 = call <vilib>:"WPI_UtilitiesGetTreeIOName.vi"("NewVal"=w395, "TreeControl in"=w397) -> ("I/O Name"=w398:string)  [unwired: 9 in]
        n192 = case shown="\"Camera\"" w398 {
          selector: w398 -> [_ w405 _ w423 w432 _]
          tunnel: w395 -> [_ _ w420 w422 _ w439]
          tunnel: w394 -> [_ _ _ _ _ w438]
          frame Default {
            w400 = FALSE ("Visible")
            w399 = FALSE ("Visible")
            n193 = property on="Motor" class="Clust (strict)"("Visible"=w399) -> ()  [unwired: 2 in, 2 out]
            n194 = property on="Ring" class="Ring (strict)"("Visible"=w399) -> ()  [unwired: 2 in, 2 out]
            n195 = property on="Rev/Fwd" class="Clust (strict)"("Visible"=w400) -> ()  [unwired: 2 in, 2 out]
            n196 = property on="On/Off" class="Bool (strict)"("Visible"=w400) -> ()  [unwired: 2 in, 2 out]
            n197 = property on="Slider" class="Slide (strict)"("Visible"=w400) -> ()  [unwired: 2 in, 2 out]
          }
          frame "Motor", "PWM" {
            w406 = FALSE ("Visible")
            n198 = case shown="\"Motor\", Default" w405 {
              tunnel: [1.0 ("Value") -1.0 ("Value")] -> w404
              tunnel: [255.0 ("Value") 1.0 ("Value")] -> w403
              tunnel: [128.0 ("Value") 0.0 ("Value")] -> w402
              tunnel: [64.0 ("Value") 0.5 ("Value")] -> w401
              frame "PWM" {
              }
              frame "Motor", Default {
              }
            }
            n199 = property on="Motor" class="Clust (strict)"("Visible"=TRUE) -> ()  [unwired: 2 in, 2 out]
            n200 = property on="Value" class="Slide (strict)"("Value"=w402, "Scale.Minimum"=w404, "Scale.Maximum"=w403, "Scale.Increment"=w401) -> ()  [unwired: 2 in, 2 out]
            n201 = property on="On/Off" class="Bool (strict)"("Visible"=w406) -> ()  [unwired: 2 in, 2 out]
            n202 = property on="Slider" class="Slide (strict)"("Visible"=w406) -> ()  [unwired: 2 in, 2 out]
            n203 = property on="Ring" class="Ring (strict)"("Visible"=w406) -> ()  [unwired: 2 in, 2 out]
            n204 = property on="Rev/Fwd" class="Clust (strict)"("Visible"=w406) -> ()  [unwired: 2 in, 2 out]
          }
          frame "Servo" {
            w418 = FALSE ("Visible")
            n205 = call <vilib>:"NT Read Number.vi"("Name"=w420) -> ("Numeric"=w419:dbl)  [unwired: 9 in, 1 out]
            n206 = property on="Slider" class="Slide (strict)"("Visible"=TRUE, "Scale.Maximum"=170.0 ("Scale.Range:Maximum")) -> ()  [unwired: 2 in, 2 out]
            n207 = local write "Slider"(w419) -> ()
            n208 = property on="Motor" class="Clust (strict)"("Visible"=w418) -> ()  [unwired: 2 in, 2 out]
            n209 = property on="Rev/Fwd" class="Clust (strict)"("Visible"=w418) -> ()  [unwired: 2 in, 2 out]
            n210 = property on="On/Off" class="Bool (strict)"("Visible"=w418) -> ()  [unwired: 2 in, 2 out]
            n211 = property on="Ring" class="Ring (strict)"("Visible"=w418) -> ()  [unwired: 2 in, 2 out]
          }
          frame "Relay", "Solenoid" {
            w421 = FALSE ("Visible")
            n212 = property on="Motor" class="Clust (strict)"("Visible"=w421) -> ()  [unwired: 2 in, 2 out]
            n213 = property on="Slider" class="Slide (strict)"("Visible"=w421) -> ()  [unwired: 2 in, 2 out]
            n214 = Search and Replace String(input string=w422, search string="/Value  **", replace string="/Direction") -> (result string=w428:string)  [unwired: 5 in, 3 out]
            n215 = property on="Ring" class="Ring (strict)"("Visible"=w421) -> ()  [unwired: 2 in, 2 out]
            n216 = call <vilib>:"NT Read String.vi"("Name"=w428) -> ("String"=w426:string)  [unwired: 9 in, 1 out]
            n217 = Equal?(x="Both directions", y=w426) -> (x = y?=w424:bool)
            n218 = Not(x=w424) -> (.not. x?=w425:bool)
            n219 = property on="Rev/Fwd" class="Clust (strict)"("Visible"=w424) -> ()  [unwired: 2 in, 2 out]
            n220 = property on="On/Off" class="Bool (strict)"("Visible"=w425, "Caption.Text"=w423) -> ()  [unwired: 2 in, 2 out]
          }
          frame "Compressor", "Digital Out" {
            w431 = FALSE ("Visible")
            # "Get direction and finish"
            n221 = property on="Motor" class="Clust (strict)"("Visible"=w431) -> ()  [unwired: 2 in, 2 out]
            n222 = property on="Slider" class="Slide (strict)"("Visible"=w431) -> ()  [unwired: 2 in, 2 out]
            n223 = property on="Ring" class="Ring (strict)"("Visible"=w431) -> ()  [unwired: 2 in, 2 out]
            n224 = property on="On/Off" class="Bool (strict)"("Visible"=TRUE, "Caption.Text"=w432) -> ()  [unwired: 2 in, 2 out]
            n225 = property on="Rev/Fwd" class="Clust (strict)"("Visible"=FALSE) -> ()  [unwired: 2 in, 2 out]
          }
          frame "Camera" {
            n226 = call <vilib>:"Get Last Path Segment.vi"("String in"=w439) -> ("String out"=w440:string)  [unwired: 10 in]
            n227 = property on="On/Off" class="Bool (strict)"("Visible"=FALSE) -> ()  [unwired: 2 in, 2 out]
            n228 = property on="Motor" class="Clust (strict)"("Visible"=FALSE) -> ()  [unwired: 2 in, 2 out]
            n229 = property on="Rev/Fwd" class="Clust (strict)"("Visible"=FALSE) -> ()  [unwired: 2 in, 2 out]
            n230 = case shown="\"White Balance  **\"" w440 {
              tunnel: w439 -> [w446 w455 w464 w473 w482 _ w488]
              tunnel: w438 -> [w444 w452 w461 w470 w479 _ _]
              frame "Size  **" {
                n231 = Index Array(array=w444) -> (element=w443:cluster{string[]})  [unwired: 1 in]
                n232 = call <vilib>:"NT Read String.vi"("Name"=w446) -> ("String"=w445:string)  [unwired: 9 in, 1 out]
                n233 = Unbundle(w443) -> (w441:string[])
                n234 = Match First String(2:w441, 3:w445) -> (0:w442:i32)  [unwired: 1 out]
                n235 = property on="Ring" class="Ring (strict)"("Value"=w442, "Strings []"=w441) -> ()  [unwired: 2 in, 2 out]
                n236 = property on="Ring" class="Ring (strict)"("Visible"=TRUE) -> ()  [unwired: 2 in, 2 out]
                n237 = property on="Slider" class="Slide (strict)"("Visible"=FALSE) -> ()  [unwired: 2 in, 2 out]
              }
              frame "White Balance  **" {
                n238 = Index Array(array=w452, index=1) -> (element=w453:cluster{string[]})
                n239 = call <vilib>:"NT Read String.vi"("Name"=w455) -> ("String"=w454:string)  [unwired: 9 in, 1 out]
                n240 = Unbundle(w453) -> (w450:string[])
                n241 = Match First String(2:w450, 3:w454) -> (0:w449:i32)  [unwired: 1 out]
                n242 = property on="Ring" class="Ring (strict)"("Value"=w449, "Strings []"=w450) -> ()  [unwired: 2 in, 2 out]
                n243 = property on="Ring" class="Ring (strict)"("Visible"=TRUE) -> ()  [unwired: 2 in, 2 out]
                n244 = property on="Slider" class="Slide (strict)"("Visible"=FALSE) -> ()  [unwired: 2 in, 2 out]
              }
              frame "Exposure  **" {
                n245 = Index Array(array=w461, index=2) -> (element=w462:cluster{string[]})
                n246 = call <vilib>:"NT Read String.vi"("Name"=w464) -> ("String"=w463:string)  [unwired: 9 in, 1 out]
                n247 = Unbundle(w462) -> (w458:string[])
                n248 = Match First String(2:w458, 3:w463) -> (0:w459:i32)  [unwired: 1 out]
                n249 = property on="Ring" class="Ring (strict)"("Value"=w459, "Strings []"=w458) -> ()  [unwired: 2 in, 2 out]
                n250 = property on="Ring" class="Ring (strict)"("Visible"=TRUE) -> ()  [unwired: 2 in, 2 out]
                n251 = property on="Slider" class="Slide (strict)"("Visible"=FALSE) -> ()  [unwired: 2 in, 2 out]
              }
              frame "Exposure Priority  **" {
                n252 = Index Array(array=w470, index=3) -> (element=w471:cluster{string[]})
                n253 = call <vilib>:"NT Read String.vi"("Name"=w473) -> ("String"=w472:string)  [unwired: 9 in, 1 out]
                n254 = Unbundle(w471) -> (w467:string[])
                n255 = Match First String(2:w467, 3:w472) -> (0:w468:i32)  [unwired: 1 out]
                n256 = property on="Ring" class="Ring (strict)"("Value"=w468, "Strings []"=w467) -> ()  [unwired: 2 in, 2 out]
                n257 = property on="Ring" class="Ring (strict)"("Visible"=TRUE) -> ()  [unwired: 2 in, 2 out]
                n258 = property on="Slider" class="Slide (strict)"("Visible"=FALSE) -> ()  [unwired: 2 in, 2 out]
              }
              frame "Color Enable  **" {
                n259 = Index Array(array=w479, index=4) -> (element=w480:cluster{string[]})
                n260 = call <vilib>:"NT Read String.vi"("Name"=w482) -> ("String"=w481:string)  [unwired: 9 in, 1 out]
                n261 = Unbundle(w480) -> (w476:string[])
                n262 = Match First String(2:w476, 3:w481) -> (0:w477:i32)  [unwired: 1 out]
                n263 = property on="Ring" class="Ring (strict)"("Value"=w477, "Strings []"=w476) -> ()  [unwired: 2 in, 2 out]
                n264 = property on="Ring" class="Ring (strict)"("Visible"=TRUE) -> ()  [unwired: 2 in, 2 out]
                n265 = property on="Slider" class="Slide (strict)"("Visible"=FALSE) -> ()  [unwired: 2 in, 2 out]
              }
              frame Default {
                n266 = property on="Ring" class="Ring (strict)"("Visible"=FALSE) -> ()  [unwired: 2 in, 2 out]
                n267 = property on="Slider" class="Slide (strict)"("Visible"=FALSE) -> ()  [unwired: 2 in, 2 out]
              }
              frame "Brightness  **", "Color Level  **", "Compression  **", "FPS  **", "Sharpness  **" {
                n268 = call <vilib>:"NT Read Number.vi"("Name"=w488) -> ("Numeric"=w487:dbl)  [unwired: 9 in, 1 out]
                n269 = local write "Slider"(w487) -> ()
                n270 = property on="Slider" class="Slide (strict)"("Visible"=TRUE, "Scale.Maximum"=100.0 ("Scale.Range:Maximum")) -> ()  [unwired: 2 in, 2 out]
                n271 = property on="Ring" class="Ring (strict)"("Visible"=FALSE) -> ()  [unwired: 2 in, 2 out]
              }
            }
          }
        }
        n272 = property on="Progress" class="Clust (strict)"("Visible"=FALSE) -> ()  [unwired: 2 in, 2 out]
      }
      event "Test Name": Mouse Enter {
        # "Populate the ring with the list of tests"
        n273 = event-data() -> ()  [unwired: 1 in, 1 out]
        n274 = call <vilib>:"NT Read String Array.vi"("Name"="TestMode/TestList") -> ("String Array"=w495:string[])  [unwired: 9 in, 1 out]
        n275 = Build Array (concatenate)("Select the test to run...", w495) -> (w494:string[])
        n276 = property on="Test Name" class="Ring (strict)"("Strings []"=w494) -> ()  [unwired: 2 in, 2 out]
      }
      event "Test Name": Value Change {
        w497 = FALSE ("Visible")
        # "Tell the robot the test name to run"
        n277 = event-data() -> ("NewVal"=w501:u16)  [unwired: 1 in]
        n278 = property on="Test Name" class="Ring (strict)"() -> ("Strings []"=w502:string[])  [unwired: 2 in, 2 out]
        n279 = local write "Progress"(T6 {"Test Progress"=0, "Test Progress Text"=""} ("Progress")) -> ()
        n280 = Index Array(array=w502, index=w501) -> (element=w500:string)
        n281 = call <vilib>:"NT Write String.vi"("String"=w500, "Name"="TestMode/TestName") -> ()  [unwired: 9 in, 1 out]
        n282 = property on="Progress" class="Clust (strict)"("Visible"=TRUE) -> ()  [unwired: 2 in, 2 out]
        n283 = property on="Motor" class="Clust (strict)"("Visible"=w497) -> ()  [unwired: 2 in, 2 out]
        n284 = property on="Slider" class="Slide (strict)"("Visible"=w497) -> ()  [unwired: 2 in, 2 out]
        n285 = property on="On/Off" class="Bool (strict)"("Visible"=w497) -> ()  [unwired: 2 in, 2 out]
        n286 = property on="Rev/Fwd" class="Clust (strict)"("Visible"=w497) -> ()  [unwired: 2 in, 2 out]
        n287 = property on="Ring" class="Ring (strict)"("Visible"=w497) -> ()  [unwired: 2 in, 2 out]
      }
      event "Listbox": Double Click {
        n288 = event-data() -> ("PlatMods.Shift"=w505:bool, "Row"=w507:i32)  [unwired: 1 in]
        n289 = case shown="False" w505 {
          tunnel: w507 -> [w511 _]
          tunnel: 1 -> [w510 _]
          frame False {
            n290 = property on="Listbox" class="LstBox (strict)"() -> ("Item Symbols"=w509:i32[])  [unwired: 2 in, 2 out]
            n291 = Replace Array Subset(array=w509, new element=w510, index=w511) -> (w508:i32[])
            n292 = property on="Listbox" class="LstBox (strict)"("Item Symbols"=w508) -> ()  [unwired: 2 in, 2 out]
          }
          frame True {
            w512 = 0 ("Top Row")
            n293 = property on="Listbox" class="LstBox (strict)"() -> ("Number of Rows"=w514:u32)  [unwired: 2 in, 2 out]
            n294 = Initialize Array(0, w514) -> (w513:i32[])
            n295 = property on="Listbox" class="LstBox (strict)"("Top Row"=w512, "Value"=w512, "Item Symbols"=w513) -> ()  [unwired: 2 in, 2 out]
          }
        }
      }
      event "Listbox": Key Down {
        n296 = event-data() -> ("VKey"=w518:T22)  [unwired: 1 in]
        n297 = case shown="\"Left\", \"Right\"" w518 {
          selector: w518 -> [w523 _]
          tunnel: eventvkey."Left" ("VKey") -> [w521 _]
          frame "Left", "Right" {
            n298 = Equal?(x=w521, y=w523) -> (x = y?=w522:bool)
            n299 = Select(t=0, s=w522, f=1) -> (s? t:f=w524:i32)
            n300 = property on="Listbox" class="LstBox (strict)"() -> ("Item Symbols"=w527:i32[])  [unwired: 2 in, 2 out]
            n301 = Replace Array Subset(array=w527, new element=w524, index="Listbox") -> (w526:i32[])
            n302 = property on="Listbox" class="LstBox (strict)"("Item Symbols"=w526) -> ()  [unwired: 2 in, 2 out]
          }
          frame Default {
          }
        }
      }
      event "DB Camera Config": Value Change {
        n303 = event-data() -> ("NewVal"=w531:bool)  [unwired: 1 in]
        n304 = case shown="False" w531 {
          tunnel: w530 -> [w540 _]
          tunnel: [w533 w551] -> w529
          tunnel: w528 -> [w532 w551]
          frame False {
            w547 = "Camera"
            w550 = FALSE ("Visible")
            n305 = local read "Camera Settings"() -> (w539:T1)
            n306 = Index Array(array=w540) -> (element=w543:cluster{string[]})  [unwired: 1 in]
            n307 = Unbundle(w539) -> ("Frate Rate"=w538:i32, "Compression"=w537:i32, "Size"=w541:u16)
            n308 = Unbundle(w543) -> (w542:string[])
            n309 = Index Array(array=w542, index=w541) -> (element=w536:string)
            n310 = call-poly <vilib>:"Write Key.vi"("section"=w547, "value"=w536, "key"="Size", "refnum"=w532) -> ("refnum out"=w549:T20)  [unwired: 2 in, 5 out]
            n311 = call-poly <vilib>:"Write Key.vi"("section"=w547, "value"=w538, "key"="FrameRate", "refnum"=w549) -> ("refnum out"=w548:T20)  [unwired: 1 in, 6 out]
            n312 = property on="Camera Settings" class="Clust (strict)"("Visible"=w550) -> ()  [unwired: 2 in, 2 out]
            n313 = local write "DB Camera Config"(w550) -> ()
            n314 = call-poly <vilib>:"Write Key.vi"("section"=w547, "value"=w537, "key"="Compression", "refnum"=w548) -> ("refnum out"=w534:T20)  [unwired: 1 in, 6 out]
            n315 = call <vilib>:"Close Config Data.vi"("refnum"=w534) -> ("file path"=w535:path)  [unwired: 2 in, 8 out]
            n316 = call <vilib>:"Open Config Data.vi"("configuration file path"=w535) -> ("refnum"=w533:T20)  [unwired: 8 in, 2 out]
          }
          frame True {
            n317 = property on="Camera Settings" class="Clust (strict)"("Visible"=TRUE) -> ()  [unwired: 2 in, 2 out]
          }
        }
      }
      event "Camera Settings": Value Change {
        n318 = event-data() -> ("NewVal"=w564:T1)  [unwired: 1 in]
        n319 = Index Array(array=w560) -> (element=w559:cluster{string[]})  [unwired: 1 in]
        n320 = Unbundle(w564) -> ("Frate Rate"=w555:i32, "Compression"=w554:i32, "Size"=w557:u16)
        n321 = Unbundle(w559) -> (w558:string[])
        n322 = Index Array(array=w558, index=w557) -> (element=w556:string)
        n323 = Format Into String(format string="%s   %dfps   %d%%", w556, w555, w554) -> (resulting string=w561:string)  [unwired: 2 in, 1 out]
        n324 = Build Array(w561) -> (w562:string[])
        n325 = property on="DB Camera Config" class="Bool (strict)"("Strings [4]"=w562) -> ()  [unwired: 2 in, 2 out]
      }
      event "Motor.Enable": Value Change {
        n326 = event-data() -> ("NewVal"=w570:bool)  [unwired: 1 in]
        n327 = Unbundle("Motor") -> ("Value"=w569:dbl)  [unwired: 1 out]
        n328 = Select(t=w569, s=w570, f=0.0) -> (s? t:f=w567:dbl)
        n329 = call <vilib>:"NT Write Number.vi"("Numeric"=w567, "Name"=w566) -> ()  [unwired: 9 in, 1 out]
      }
      event "Slider": Value Change {
        n330 = event-data() -> ("NewVal"=w573:dbl)  [unwired: 1 in]
        n331 = call <vilib>:"NT Write Number.vi"("Numeric"=w573, "Name"=w574) -> ()  [unwired: 9 in, 1 out]
      }
      event "On/Off": Value Change {
        n332 = event-data() -> ("NewVal"=w578:bool)  [unwired: 1 in]
        n333 = Boolean To (0,1)(Boolean=w578) -> (0, 1=w577:i16)
        n334 = call <vilib>:"NT Write Number.vi"("Numeric"=w577, "Name"=w576) -> ()  [unwired: 9 in, 1 out]
      }
      event "Rev/Fwd": Value Change {
        n335 = event-data() -> ("NewVal.Forward"=w586:bool, "NewVal.Reverse"=w585:bool)  [unwired: 1 in]
        n336 = Boolean To (0,1)(Boolean=w586) -> (0, 1=w582:i16)
        n337 = Boolean To (0,1)(Boolean=w585) -> (0, 1=w584:i16)
        n338 = Negate(x=w584) -> (-x=w583:i16)
        n339 = Add(x=w582, y=w583) -> (x+y=w581:i16)
        n340 = call <vilib>:"NT Write Number.vi"("Numeric"=w581, "Name"=w580) -> ()  [unwired: 9 in, 1 out]
      }
      event "Ring": Value Change {
        n341 = event-data() -> ("NewVal"=w590:u16)  [unwired: 1 in]
        n342 = property on="Ring" class="Ring (strict)"() -> ("Strings []"=w591:string[])  [unwired: 2 in, 2 out]
        n343 = Index Array(array=w591, index=w590) -> (element=w589:string)
        n344 = call <vilib>:"NT Write String.vi"("String"=w589, "Name"=w588) -> ()  [unwired: 9 in, 1 out]
      }
    }
  }
  n345 = Index Array(array=w19) -> (element=w20:cluster{string[]})  [unwired: 1 in]
  n346 = Unbundle(w20) -> (w18:string[])
  n347 = Match First String(2:w18, 3:w17) -> (0:w16:i32)  [unwired: 1 out]
  n348 = Bundle("value"=w22, "value"=w21, "index"=w16) -> (w10:cluster{"value":i32, "value":i32, "index":i32})  [unwired: 1 out]
  n349 = property on="On/Off" class="Bool (strict)"("Visible"=w33) -> ()  [unwired: 2 in, 2 out]
  n350 = property on="Motor" class="Clust (strict)"("Visible"=w33) -> ()  [unwired: 2 in, 2 out]
  n351 = property on="Progress" class="Clust (strict)"("Visible"=w33) -> ()  [unwired: 2 in, 2 out]
  n352 = property on="Ring" class="Ring (strict)"("Visible"=w33) -> ()  [unwired: 2 in, 2 out]
  n353 = property on="Camera Settings" class="Clust (strict)"("Val(Sgnl)"=w10) -> ()  [unwired: 2 in, 2 out]
  n354 = property on="Rev/Fwd" class="Clust (strict)"("Visible"=w33) -> ()  [unwired: 2 in, 2 out]
  n355 = property on="Camera Settings" class="Clust (strict)"("Visible"=w33) -> ()  [unwired: 2 in, 2 out]
  n356 = local write "DB Camera Config"(w33) -> ()
